vi "get ambient light level.vi"(8 "error in":errorcluster) -> (0 "error out":errorcluster, 2 "light level":u8)   [LabVIEW 2013]
uses:
  <vilib>/myRIO/Instrument Drivers/Onboard IO/DIO/vis/Smart Open.vi
  <vilib>/myRIO/Instrument Drivers/Onboard IO/DIO/vis/Write.vi
  <vilib>/myRIO/Instrument Drivers/Onboard IO/SPI/vis/Smart Open.vi
  <vilib>/myRIO/Instrument Drivers/Onboard IO/SPI/vis/Configure.vi
  <vilib>/myRIO/Instrument Drivers/Onboard IO/SPI/vis/Read.vi
  <vilib>/myRIO/Instrument Drivers/Onboard IO/DIO/vis/Open.vi
  <vilib>/myRIO/Instrument Drivers/Onboard IO/SPI/vis/Open.vi
  <vilib>/myRIO/Instrument Drivers/Onboard IO/SPI/vis/Write Read.vi
  <vilib>/myRIO/Common/Instrument Driver Framework/myRIO v1.0/DIO/vis/myRIO v1.1 Open DIO.vi
  <vilib>/myRIO/Common/Instrument Driver Framework/myRIO v1.0/SPI/vis/myRIO v1.1 Open SPI.vi
  <vilib>/myRIO/Common/Instrument Driver Framework/Utilities/vis/Validate Channels.vi
  <vilib>/myRIO/Common/Instrument Driver Framework/myRIO v1.0/DIO/vis/myRIO v1.0 Reserve DIO.vi
  <vilib>/myRIO/Common/Instrument Driver Framework/myRIO v1.0/SPI/vis/myRIO v1.0 Reserve SPI.vi
  <vilib>/myRIO/Common/Instrument Driver Framework/myRIO v1.0/Resource Manager/vis/myRIO v1.0 Reserve Channel List.vi
  <vilib>/myRIO/Common/Instrument Driver Framework/myRIO v1.0/DIO/vis/myRIO v1.0 Build MUX Configuration DIO.vi
  <vilib>/myRIO/Common/Instrument Driver Framework/myRIO v1.0/SPI/vis/myRIO v1.0 Build MUX Configuration SPI.vi
  <vilib>/myRIO/Common/Instrument Driver Framework/myRIO v1.0/Resource Manager/vis/myRIO v1.0 Reserve Channel.vi
  <vilib>/myRIO/Common/Instrument Driver Framework/myRIO v1.0/Resource Manager/vis/myRIO v1.0 Unreserve Channel.vi
  <vilib>/myRIO/Common/Instrument Driver Framework/myRIO v1.0/Resource Manager/vis/myRIO v1.0 Create Configuration List.vi
  <vilib>/myRIO/Common/Instrument Driver Framework/myRIO v1.0/Resource Manager/vis/myRIO v1.0 Build Mutex Name.vi
  <vilib>/myRIO/Common/Instrument Driver Framework/myRIO v1.0/myRIO v1.1 Open.vi
  <vilib>/Utility/VariantDataType/GetNumericInfo.vi
  <vilib>/Utility/error.llb/Error Cluster From Error Code.vi
  <vilib>/myRIO/Common/Instrument Driver Framework/Utilities/vis/IO Manager.vi
  <vilib>/myRIO/Common/Instrument Driver Framework/Utilities/vis/Configuration Manager.vi
  <vilib>/myRIO/Common/Instrument Driver Framework/myRIO v1.0/Resource Manager/vis/myRIO v1.0 Configure IO.vi
  <vilib>/myRIO/Common/Instrument Driver Framework/myRIO v1.0/myRIO v1.0 Close.vi
  <vilib>/myRIO/Common/Instrument Driver Framework/myRIO v1.0/DIO/vis/myRIO v1.0 Write DIO.vi
  <vilib>/myRIO/Common/Instrument Driver Framework/myRIO v1.0/SPI/vis/myRIO v1.0 Configure SPI.vi
  <vilib>/myRIO/Common/Instrument Driver Framework/myRIO v1.0/SPI/vis/myRIO v1.0 Write Read SPI.vi
panel:
  # "get ambient light level"
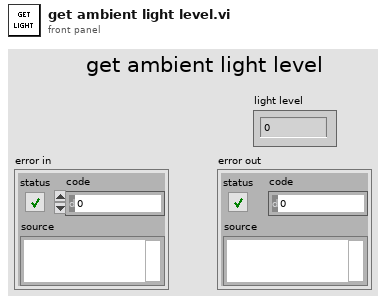
[diagram p1: front panel]
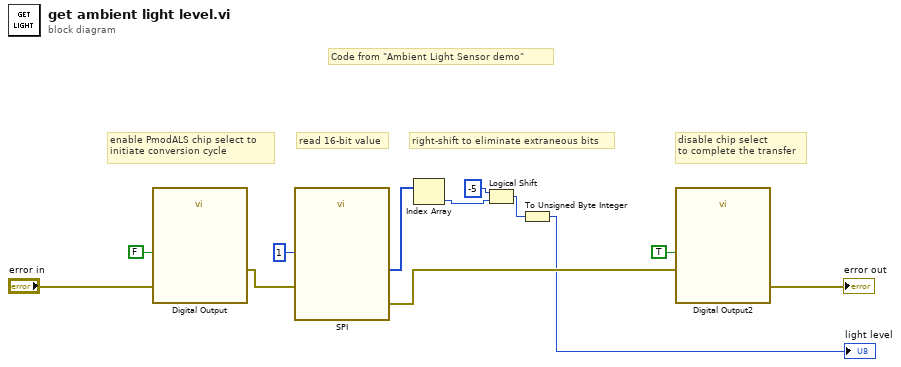
[diagram p0: block diagram]
diagram:
  # "Code from \"Ambient Light Sensor demo\""
  # "right-shift to eliminate extraneous bits"
  # "disable chip select\nto complete the transfer"
  # "read 16-bit value"
  # "enable PmodALS chip select to\ninitiate conversion cycle"
  n1 = call "Digital Output"("B/DIO0 (Pin 11)"=FALSE ("A/DIO0 (Pin 11)"), "error in (no error)"="error in") -> ("error out"=w11:errorcluster)  [unwired: 25 in]
  n2 = call "SPI"("Frame Count"=u32 1, "error in (no error)"=w11) -> ("Frames Read"=w7:u16[], "error out"=w9:errorcluster)  [unwired: 24 in]
  n3 = Index Array "Index Array"(array=w7) -> (element=w6:u16)  [unwired: 1 in]
  n4 = Logical Shift(y=i16 -5, x=w6) -> (x << y=w4:u16)
  n5 = To Unsigned Byte Integer(number=w4) -> (unsigned 8bit integer=→"light level":u8)
  n6 = call "Digital Output2"("B/DIO0 (Pin 11)"=TRUE ("A/DIO0 (Pin 11)"), "error in (no error)"=w9) -> ("error out"=→"error out":errorcluster)  [unwired: 25 in]
